vi "Logger DVR FGV.vi"(7 "FGV Actions":T1=enum."Get", 8 "error in":errorcluster, 11 "Logger in":refnum<class "Logger.lvclass">) -> (0 "error out":errorcluster, 3 "Logger DVR":refnum<data-value>)   [LabVIEW 2024, in "hse-logger.lvlib"]
doc: "This FGV stores a reference (DVR) to a Logger object. \nThe default action is to *get* the DVR (if you do not wire a ``FGV_Actions`` control).\n\n____\nHAMPEL SOFTWARE ENGINEERING v2.2.2 (2025-01-16 15:41)"
uses:
  <vilib>/Hampel Software Engineering/HSE Logger/hse-logger.lvlib
  <vilib>/Hampel Software Engineering/HSE Logger/Logger/Logger.lvclass
  <vilib>/Hampel Software Engineering/HSE Logger/FGV Actions.ctl
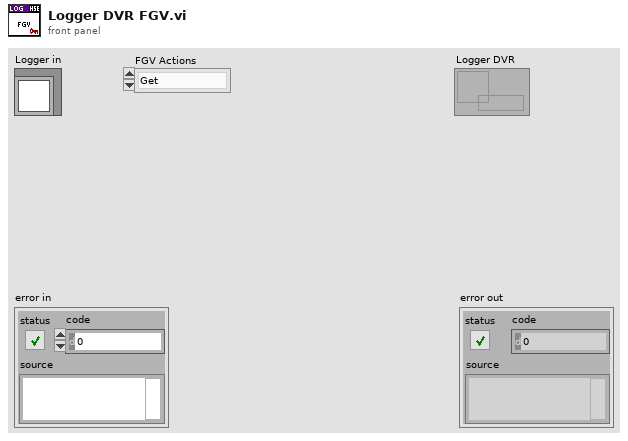
[diagram p1: front panel]
types:
  T1 = typedef "hse-logger.lvlib/FGV Actions.ctl" = enum16{"Set", "Get"}
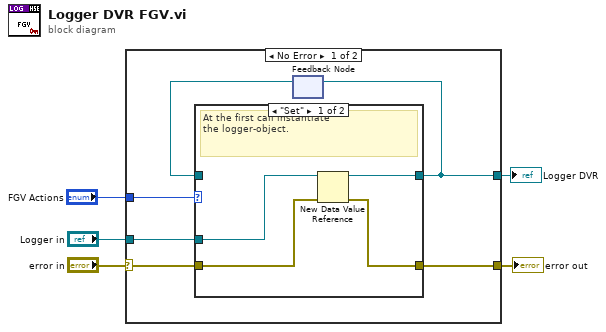
[diagram p0: block diagram]
diagram:
  n1 = case shown="No Error" "error in" {
    selector: "error in" -> [w9 w18]
    tunnel: [w7 _] -> w4
    tunnel: [w11 w18] -> w3
    tunnel: "Logger in" -> [w10 _]
    tunnel: "FGV Actions" -> [w8 _]
    frame No Error {
      n2 = feedback #1() -> (w6:refnum<data-value>)  [unwired: 1 in]
      n3 = case shown="\"Set\"" w8 {
        tunnel: [w15 w17] -> w7
        tunnel: w6 -> [_ w17]
        tunnel: [w13 w16] -> w11
        tunnel: w10 -> [w14 _]
        tunnel: w9 -> [w12 w16]
        frame "Set" {
          # "At the first call instantiate\nthe logger-object."
          n4 = New Data Value Reference(data value=w14, error in=w12) -> (data value reference=w15:refnum<data-value>, error out=w13:errorcluster)
        }
        frame "Get", Default {
          # "Reference already in shift register."
        }
      }
      n5 = feedback-in #1(w7) -> ()
    }
    frame Error {
    }
  }
  "error out" <- w3
  "Logger DVR" <- w4
